vi "Open Audio File Write.vi"   [LabVIEW 2020, in "G-Audio.lvlib"]
doc: "Opens an audio file and initializes the relevant encoder. Codec specific settings are wired to the <b>Codec Specific Info</b> input.\n\nSupported codecs: wav"
uses:
  G-Audio.lvlib
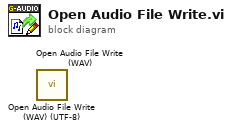
[diagram p0: block diagram]
diagram:
  n1 = call "Open Audio File Write (WAV) (UTF-8).vi"() -> ()  [unwired: 10 in, 2 out]
  n2 = call "Open Audio File Write (WAV).vi"() -> ()  [unwired: 10 in, 2 out]
